vi "Command.Diagnostic Data Lookup Table.vi"(5 "Command Refs":T2, 6 "command":T3=enum."Get All", 7 "Name":string, 8 "error in (no error)":errorcluster {"code" min=0 max=0}, 9 "Signals":dbl[](array[numeric]), 10 "Signal In":dbl, 11 "Diag Data Ref":T1) -> (0 "error out":errorcluster {"code" min=0 max=0}, 1 "Signals Out":dbl[](array[numeric]), 2 "Signal Out":dbl, 3 "Diag Data Ref out":T1)   [LabVIEW 2015, in "J1939 Addon Engine.lvlib"]
uses:
  J1939 Addon Engine.lvlib
  Types/Command.Diagnostic Data Lookup Table Action.ctl
  Types/Command.Configuration.ctl
  Types/Command.Diagnostic Data Lookup Table Reference.ctl
  Types/Command.Diagnostic Data Lookup Table State Variables.ctl
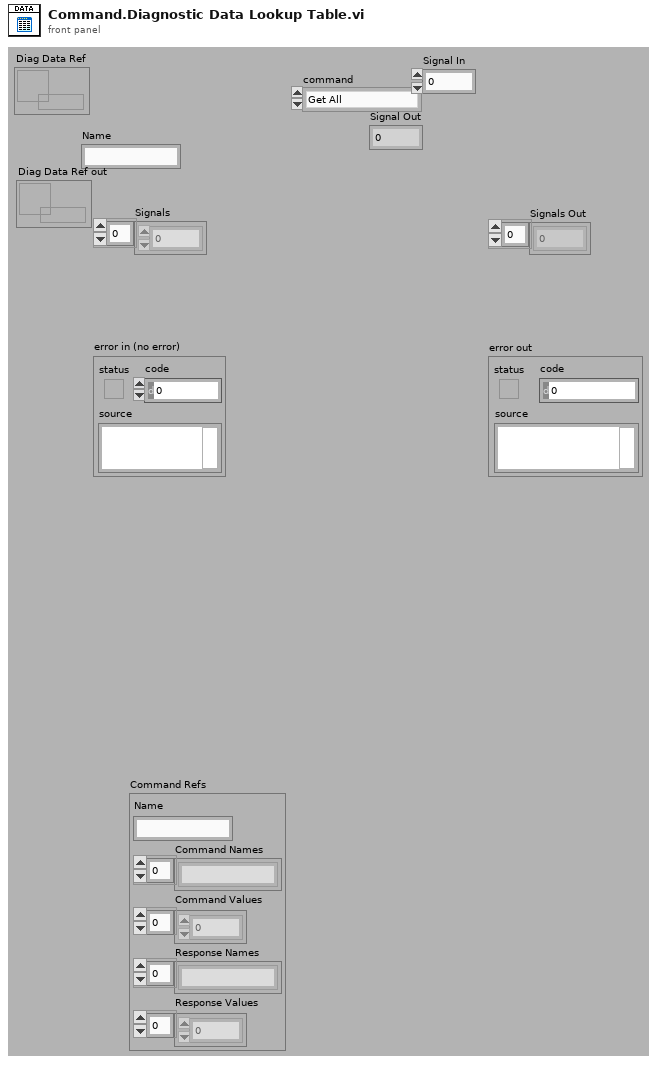
[diagram p1: front panel]
types:
  T1 = typedef "J1939 Addon Engine.lvlib/Command.Diagnostic Data Lookup Table Reference.ctl" = refnum<data-value>
  T2 = typedef "J1939 Addon Engine.lvlib/Command.Configuration.ctl" = cluster{"Name":string, "Command Names":string[], "Command Values":dbl[], "Response Names":string[], "Response Values":dbl[]}
  T3 = typedef "J1939 Addon Engine.lvlib/Command.Diagnostic Data Lookup Table Action.ctl" = enum16{"Initialize", "Get All", "Set All", "Set Value", "Get Value"}
  T4 = typedef "J1939 Addon Engine.lvlib/Command.Diagnostic Data Lookup Table State Variables.ctl" = cluster{"LUT":variant, "Response Names":string[], "Command Names":string[]}
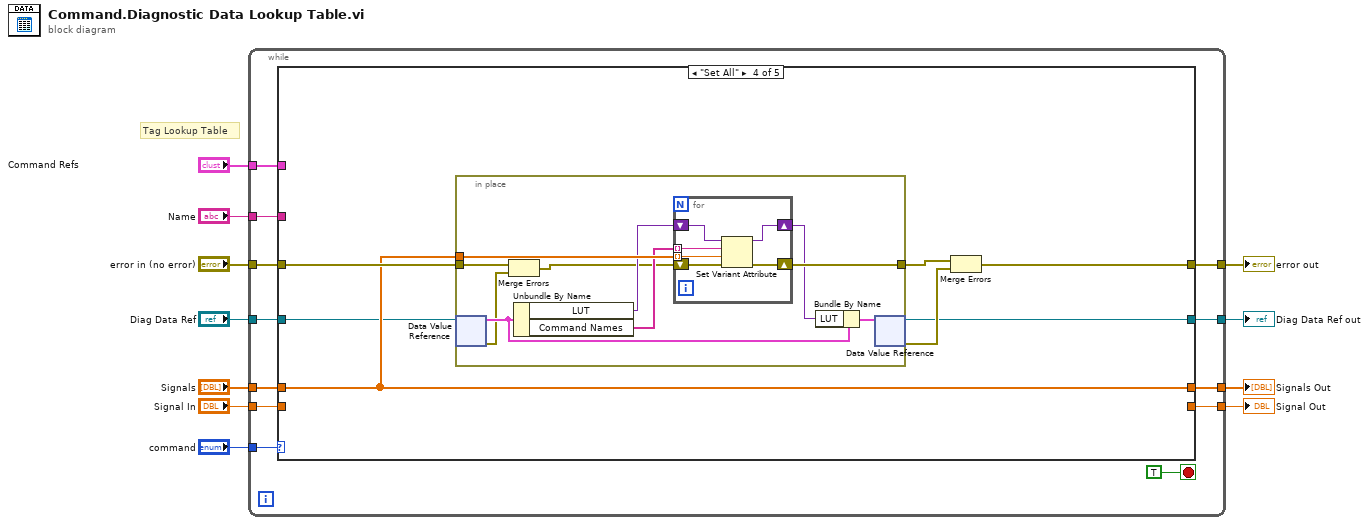
[diagram p0: block diagram]
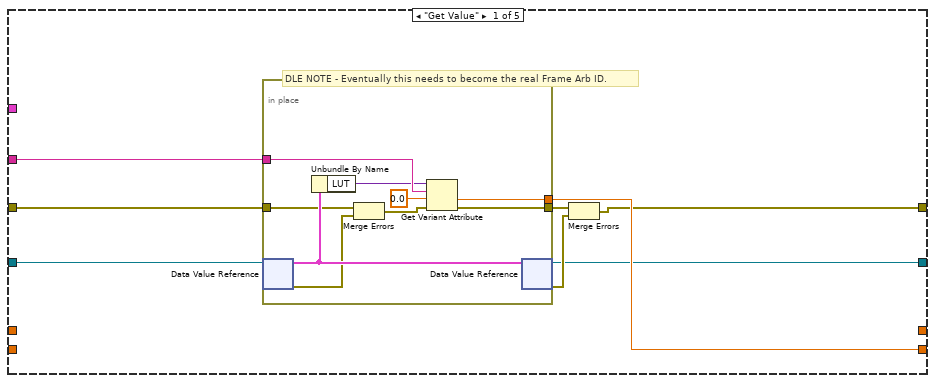
[diagram p2: hidden frame]
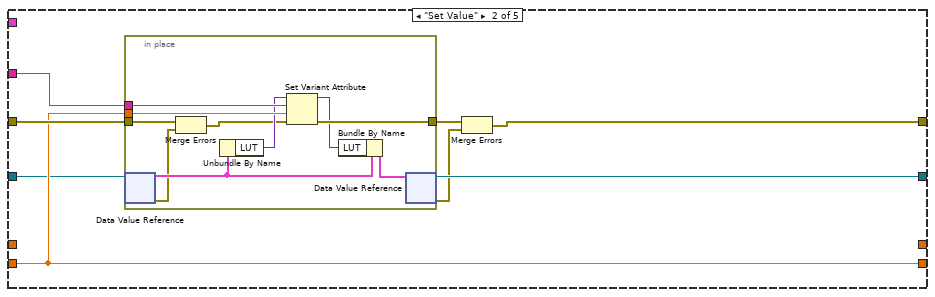
[diagram p3: hidden frame]
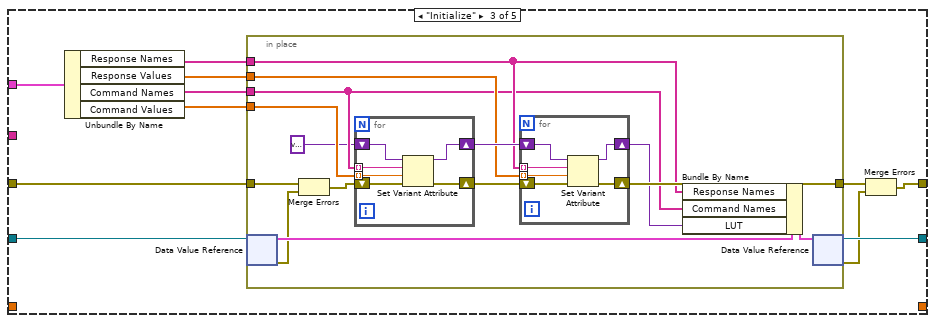
[diagram p4: hidden frame]
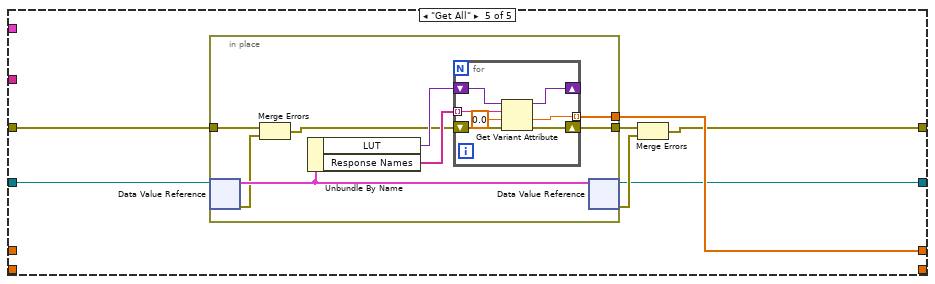
[diagram p5: hidden frame]
diagram:
  # "Tag Lookup Table"
  n1 = while {
    tunnel: "command" -> [w22]
    tunnel: "error in (no error)" -> [w21]
    tunnel: [w20] -> w9
    tunnel: "Name" -> [w19]
    tunnel: "Command Refs" -> [w18]
    tunnel: [w17] -> w5
    tunnel: "Signals" -> [w16]
    tunnel: [w15] -> w4
    tunnel: "Signal In" -> [w14]
    tunnel: "Diag Data Ref" -> [w13]
    tunnel: [w12] -> w1
    stop <- TRUE stop-if-true
    n2 = case shown="\"Set All\"" w22 {
      tunnel: w21 -> [w31 w48 w69 w102 w125]
      tunnel: [w26 w42 w60 w98 w121] -> w20
      tunnel: w19 -> [w30 w47 _ _ _]
      tunnel: w18 -> [_ _ w68 _ _]
      tunnel: [_ _ _ w101 w124] -> w17
      tunnel: w16 -> [_ _ _ w101 _]
      tunnel: [w29 w46 _ _ _] -> w15
      tunnel: w14 -> [_ w46 _ _ _]
      tunnel: w13 -> [w28 w45 w63 w100 w123]
      tunnel: [w24 w44 w62 w96 w119] -> w12
      frame "Get Value" {
        # "DLE NOTE - Eventually this needs to become the real Frame Arb ID."
        n3 = in-place {
          in-place-border: w31 -> [w33]
          in-place-border: [w40] -> w25
          in-place-border: w30 -> [w38]
          in-place-border: [w37] -> w29
          n4 = in-place-dvr #1(w28) -> (w35:T4, w34:errorcluster)
          n5 = Unbundle By Name(w35) -> ("LUT"=w36:variant)
          n6 = Merge Errors(w33, w34) -> (w32:errorcluster)
          n7 = Get Variant Attribute(Variant=w36, name=w38, default value (empty Variant)=0.0, error in=w32) -> (value=w37:dbl, error out=w40:errorcluster)  [unwired: 2 out]
          n8 = in-place-dvr #1(w35) -> (w24:T1, w27:errorcluster)
        }
        n9 = Merge Errors(w25, w27) -> (w26:errorcluster)
      }
      frame "Set Value" {
        n10 = in-place {
          in-place-border: w48 -> [w58]
          in-place-border: [w57] -> w41
          in-place-border: w47 -> [w56]
          in-place-border: w46 -> [w55]
          n11 = in-place-dvr #2(w45) -> (w53:T4, w49:errorcluster)
          n12 = Merge Errors(w58, w49) -> (w50:errorcluster)
          n13 = Unbundle By Name(w53) -> ("LUT"=w54:variant)
          n14 = Set Variant Attribute(Variant=w54, name=w56, value=w55, error in=w50) -> (Variant out=w51:variant, error out=w57:errorcluster)  [unwired: 1 out]
          n15 = Bundle By Name(cluster=w53, "LUT"=w51) -> (w52:T4)
          n16 = in-place-dvr #2(w52) -> (w44:T1, w43:errorcluster)
        }
        n17 = Merge Errors(w41, w43) -> (w42:errorcluster)
      }
      frame "Initialize" {
        n18 = Unbundle By Name(w68) -> ("Response Names"=w65:string[], "Response Values"=w66:dbl[], "Command Names"=w64:string[], "Command Values"=w67:dbl[])
        n19 = in-place {
          in-place-border: w69 -> [w72]
          in-place-border: [w81] -> w59
          in-place-border: w67 -> [w80]
          in-place-border: w66 -> [w79]
          in-place-border: w65 -> [w76]
          in-place-border: w64 -> [w75]
          n20 = in-place-dvr #3(w63) -> (w78:T4, w73:errorcluster)
          n21 = Merge Errors(w72, w73) -> (w71:errorcluster)
          n22 = for {
            shift-right: [w94] -> w82
            shift-left: variant ("LUT") -> [w95]
            shift-right: [w92] -> w83
            shift-left: w71 -> [w93]
            tunnel: w75 -> [w91] mode=indexing
            tunnel: w80 -> [w90] mode=indexing
            n23 = Set Variant Attribute(Variant=w95, name=w91, value=w90, error in=w93) -> (Variant out=w94:variant, error out=w92:errorcluster)  [unwired: 1 out]
          }
          n24 = for {
            shift-right: [w88] -> w77
            shift-left: w82 -> [w89]
            shift-right: [w86] -> w81
            shift-left: w83 -> [w87]
            tunnel: w79 -> [w85] mode=indexing
            tunnel: w76 -> [w84] mode=indexing
            n25 = Set Variant Attribute(Variant=w89, name=w84, value=w85, error in=w87) -> (Variant out=w88:variant, error out=w86:errorcluster)  [unwired: 1 out]
          }
          n26 = Bundle By Name(cluster=w78, "Response Names"=w76, "Command Names"=w75, "LUT"=w77) -> (w74:T4)
          n27 = in-place-dvr #3(w74) -> (w62:T1, w61:errorcluster)
        }
        n28 = Merge Errors(w59, w61) -> (w60:errorcluster)
      }
      frame "Set All" {
        n29 = in-place {
          in-place-border: [w112] -> w97
          in-place-border: w102 -> [w104]
          in-place-border: w101 -> [w111]
          n30 = in-place-dvr #4(w100) -> (w108:T4, w105:errorcluster)
          n31 = Merge Errors(w104, w105) -> (w103:errorcluster)
          n32 = Unbundle By Name(w108) -> ("LUT"=w110:variant, "Command Names"=w109:string[])
          n33 = for {
            shift-right: [w117] -> w107
            shift-left: w110 -> [w118]
            shift-right: [w115] -> w112
            shift-left: w103 -> [w116]
            tunnel: w111 -> [w114] mode=indexing
            tunnel: w109 -> [w113] mode=indexing
            n34 = Set Variant Attribute(Variant=w118, name=w113, value=w114, error in=w116) -> (Variant out=w117:variant, error out=w115:errorcluster)  [unwired: 1 out]
          }
          n35 = Bundle By Name(cluster=w108, "LUT"=w107) -> (w106:T4)
          n36 = in-place-dvr #4(w106) -> (w96:T1, w99:errorcluster)
        }
        n37 = Merge Errors(w97, w99) -> (w98:errorcluster)
      }
      frame "Get All" {
        n38 = in-place {
          in-place-border: w125 -> [w127]
          in-place-border: [w133] -> w120
          in-place-border: [w132] -> w124
          n39 = in-place-dvr #5(w123) -> (w129:T4, w128:errorcluster)
          n40 = Merge Errors(w127, w128) -> (w126:errorcluster)
          n41 = Unbundle By Name(w129) -> ("LUT"=w131:variant, "Response Names"=w130:string[])
          n42 = for {
            shift-right: [w139] -> _
            shift-left: w131 -> [w140]
            shift-right: [w137] -> w133
            shift-left: w126 -> [w138]
            tunnel: w130 -> [w136] mode=indexing
            tunnel: [w134] -> w132 mode=indexing
            n43 = Get Variant Attribute(Variant=w140, name=w136, default value (empty Variant)=0.0, error in=w138) -> (duplicate Variant=w139:variant, value=w134:dbl, error out=w137:errorcluster)  [unwired: 1 out]
          }
          n44 = in-place-dvr #5(w129) -> (w119:T1, w122:errorcluster)
        }
        n45 = Merge Errors(w120, w122) -> (w121:errorcluster)
      }
    }
  }
  "error out" <- w9
  "Signals Out" <- w5
  "Signal Out" <- w4
  "Diag Data Ref out" <- w1
